vi "UpdateDeviceList.vi"(8 "error in (no error)":errorcluster, 9 "Section List":string[](array[string]), 10 "Device":u16(ring), 11 "Device List":refnum<k7>) -> (0 "error out":errorcluster, 1 "New Section List":string[](array[string]), 2 "New Label List":string[](array[string]), 3 "New Device Index":i32)   [LabVIEW 2016]
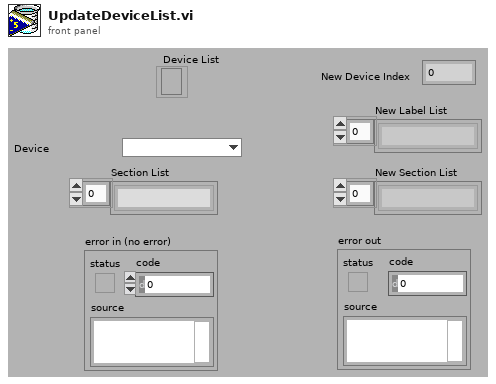
[diagram p1: front panel]
types:
  T1 = cluster{"status":bool, "code":u32, "source":string}
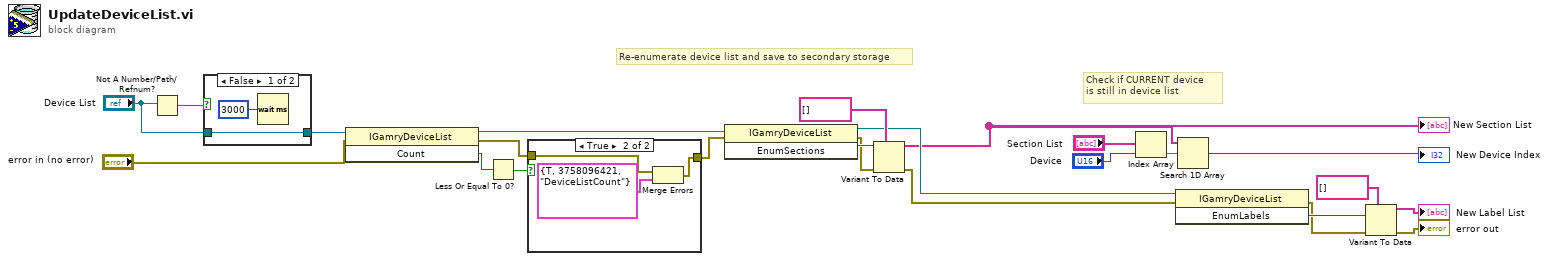
[diagram p0: block diagram]
diagram:
  # "Check if CURRENT device\nis still in device list"
  # "Re-enumerate device list and save to secondary storage"
  n1 = Not A Number/Path/Refnum?(number/path/refnum="Device List") -> (NaN/Path/Refnum?=w10:bool)
  n2 = case shown="False" w10 {
    tunnel: [w25 w27] -> w9
    tunnel: "Device List" -> [w25 w27]
    frame False {
      n3 = Wait (ms)(milliseconds to wait=u32 3000) -> ()  [unwired: 1 out]
    }
    frame True {
    }
  }
  n4 = invoke class="IGamryDeviceList" method="Count"(reference=w9, error in="error in (no error)") -> (reference out=w14:refnum<k7>, error out=w17:errorcluster, "Count"=w20:i32)  [unwired: 1 in]
  n5 = Less Or Equal To 0?(x=w20) -> (x <= 0?=w18:bool)
  n6 = case shown="True" w18 {
    tunnel: [w28 w31] -> w15
    tunnel: w17 -> [w28 w29]
    frame False {
    }
    frame True {
      n7 = Merge Errors(w29, T1 {"status"=TRUE, "code"=3758096421, "source"="DeviceListCount"} ("error out")) -> (w31:errorcluster)
    }
  }
  n8 = invoke class="IGamryDeviceList" method="EnumSections"(reference=w14, error in=w15) -> (reference out=w11:refnum<k7>, error out=w19:errorcluster, "EnumSections"=w24:variant)  [unwired: 1 in]
  n9 = Variant To Data(error in=w19, type=string[] [], Variant=w24) -> (data=w5:string[], error out=w12:errorcluster)
  "New Section List" <- w5
  n10 = Index Array(array="Section List", index="Device") -> (element=w21:string)
  n11 = invoke class="IGamryDeviceList" method="EnumLabels"(reference=w11, error in=w12) -> (error out=w13:errorcluster, "EnumLabels"=w22:variant)  [unwired: 1 in, 1 out]
  n12 = Search 1D Array(1D array=w5, element=w21) -> (index of element=→"New Device Index":i32)  [unwired: 1 in]
  n13 = Variant To Data(error in=w13, type=string[] [], Variant=w22) -> (data=→"New Label List":string[], error out=→"error out":errorcluster)
